vi "SRV_VIG_System Config-Enable Diagnostic Logging.vi"(7 "Enable Diagnostic Log":bool, 12 "Method (Get)":enum16{"Get", "Set"}(ring)) -> (8 "Enable Diagnostic Log?":bool)   [LabVIEW 2014]
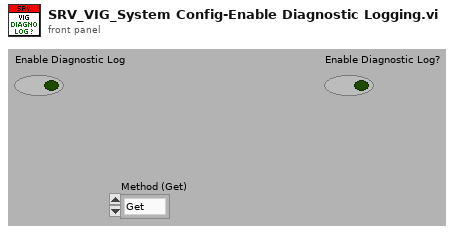
[diagram p1: front panel]
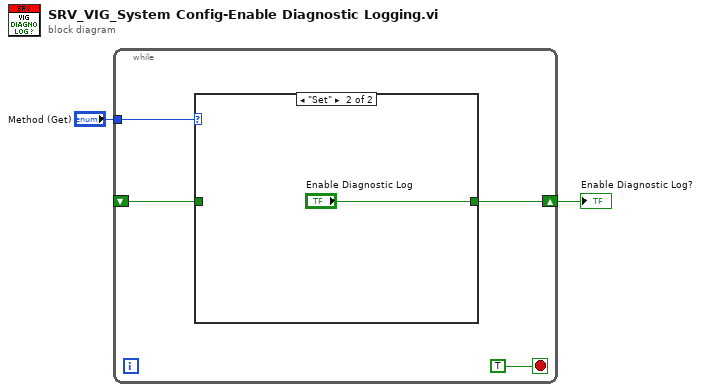
[diagram p0: block diagram]
diagram:
  n1 = while {
    tunnel: "Method (Get)" -> [w6]
    shift-right: [w4] -> w1
    shift-left: _ -> [w5]
    stop <- TRUE stop-if-true
    n2 = case shown="\"Set\"" w6 {
      tunnel: w5 -> [w7 _]
      tunnel: [w7 "Enable Diagnostic Log"] -> w4
      frame "Get" {
      }
      frame "Set" {
      }
    }
  }
  "Enable Diagnostic Log?" <- w1
